vi "Debug - Initialize.vi"(7 "Debug Mode":bool, 8 "error in (no error)":errorcluster, 11 "Packet Name":string) -> (0 "error out":errorcluster, 3 "Debug Log File":refnum<file>)   [LabVIEW 2021, in "UDP-Custom-Device Engine.lvlib"]
uses:
  UDP-Custom-Device Engine.lvlib
  <vilib>/NI VeriStand/Custom Device Tools/Custom Device Utility Library/Custom Device Utility Library.lvlib
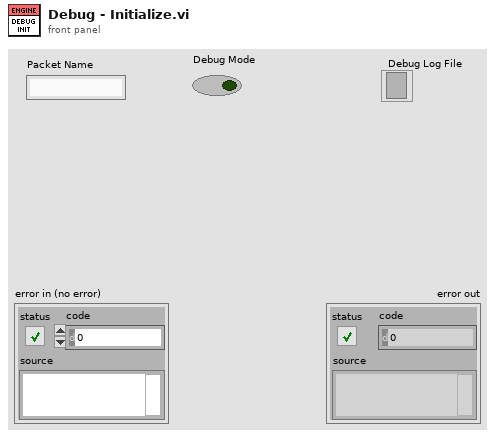
[diagram p1: front panel]
types:
  T1 = enum16{"open", "replace", "create", "open or create", "replace or create", "replace or create with confirmation"}
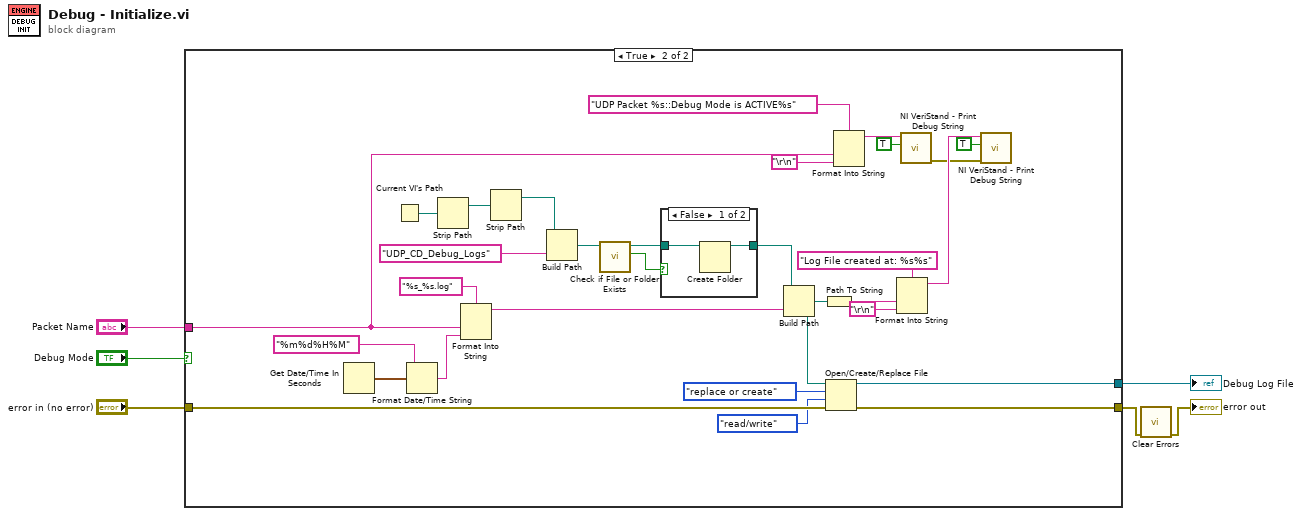
[diagram p0: block diagram]
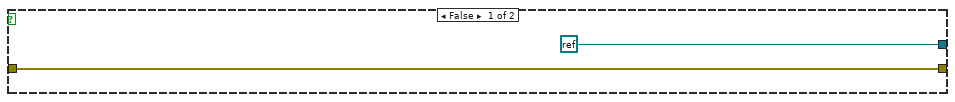
[diagram p2: hidden frame]
diagram:
  n1 = case shown="True" "Debug Mode" {
    tunnel: [w8 w38] -> w1
    tunnel: "error in (no error)" -> [w8 w37]
    tunnel: "Packet Name" -> [_ w18]
    tunnel: [refnum<k0> refnum w36] -> w4
    frame False {
    }
    frame True {
      n2 = Get Date/Time In Seconds() -> (seconds since 1Jan1904=w23:timestamp)
      n3 = Current VI's Path() -> (path=w29:path)
      n4 = Format Date/Time String(time format string (%c)="%m%d%H%M", seconds (now)=w23) -> (date/time string=w22:string)  [unwired: 1 in]
      n5 = Strip Path(path=w29) -> (stripped path=w28:path)  [unwired: 1 out]
      n6 = Format Into String(format string="%s_%s.log", w18, w22) -> (resulting string=w34:string)  [unwired: 2 in, 1 out]
      n7 = Strip Path(path=w28) -> (stripped path=w30:path)  [unwired: 1 out]
      n8 = Build Path(base path=w30, name or relative path="UDP_CD_Debug_Logs") -> (appended path=w27:path)
      n9 = call <vilib>:"Check if File or Folder Exists.vi"("path"=w27) -> ("file or folder exists?"=w24:bool, "dup path"=w26:path)  [unwired: 8 in, 1 out]
      n10 = case shown="False" w24 {
        tunnel: w26 -> [w40 w41]
        tunnel: [w39 w41] -> w25
        frame False {
          n11 = Create Folder(path (use dialog)=w40) -> (created path=w39:path)  [unwired: 2 in, 2 out]
        }
        frame True {
        }
      }
      n12 = Build Path(base path=w25, name or relative path=w34) -> (appended path=w13:path)
      n13 = Path To String(path=w13) -> (string=w12:string)
      n14 = Open/Create/Replace File(file path (use dialog)=w13, error in=w37, operation (0:open)=T1."replace or create", access (0:read/write)=enum16{"read/write", "read-only", "write-only"}."read/write") -> (refnum out=w36:refnum<file>, error out=w38:errorcluster)  [unwired: 2 in, 1 out]
      n15 = Format Into String(format string="UDP Packet %s::Debug Mode is ACTIVE%s", w18, "\r\n") -> (resulting string=w16:string)  [unwired: 2 in, 1 out]
      n16 = Format Into String(format string="Log File created at: %s%s", w12, "\r\n") -> (resulting string=w10:string)  [unwired: 2 in, 1 out]
      n17 = call <vilib>:"NI VeriStand - Print Debug String.vi"("Add to log file? (F)"=TRUE ("Add to log file? (T)"), "Message"=w16) -> ("error out"=w9:errorcluster)  [unwired: 9 in]
      n18 = call <vilib>:"NI VeriStand - Print Debug String.vi"("error in (no error)"=w9, "Add to log file? (F)"=TRUE ("Add to log file? (T)"), "Message"=w10) -> ()  [unwired: 8 in, 1 out]
    }
  }
  "Debug Log File" <- w4
  n19 = call <vilib>:"Clear Errors.vi"("error in (no error)"=w1) -> ("error out"=→"error out":errorcluster)  [unwired: 5 in, 1 out]
